vi "Constants.vi"() -> ()   [LabVIEW 2016, in "UDP CD Shared.lvlib"]
doc: "Use this Global VI to access the GUIDs assigned to the page resources of the Custom Device."
uses:
  UDP CD Shared.lvlib
panel:
  in  "Tab Control":enum32{"GUIDS", "Constants", "Properties"}(tab)
  in  "UDP CD":string="0fecbe6b-c3c3-4526-8850-50f5321f642f"
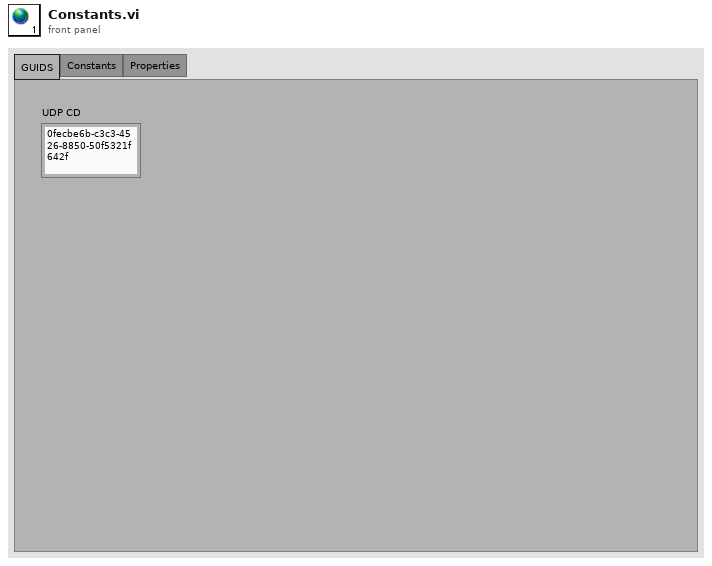
[diagram p1: front panel]
diagram:
